vi "Example.vi"() -> ()   [LabVIEW 2019, in "Database_Postgress.lvclass"]
uses:
  Database_Postgress.lvclass
  Query Return.ctl
  Connection Info.ctl
  DatabaseInterface_class/DatabaseInterface.lvclass
panel:
  in  "Query":string="SELECT version();"
  out "Query Return":T1[](array[typedef])
  out "error out":errorcluster
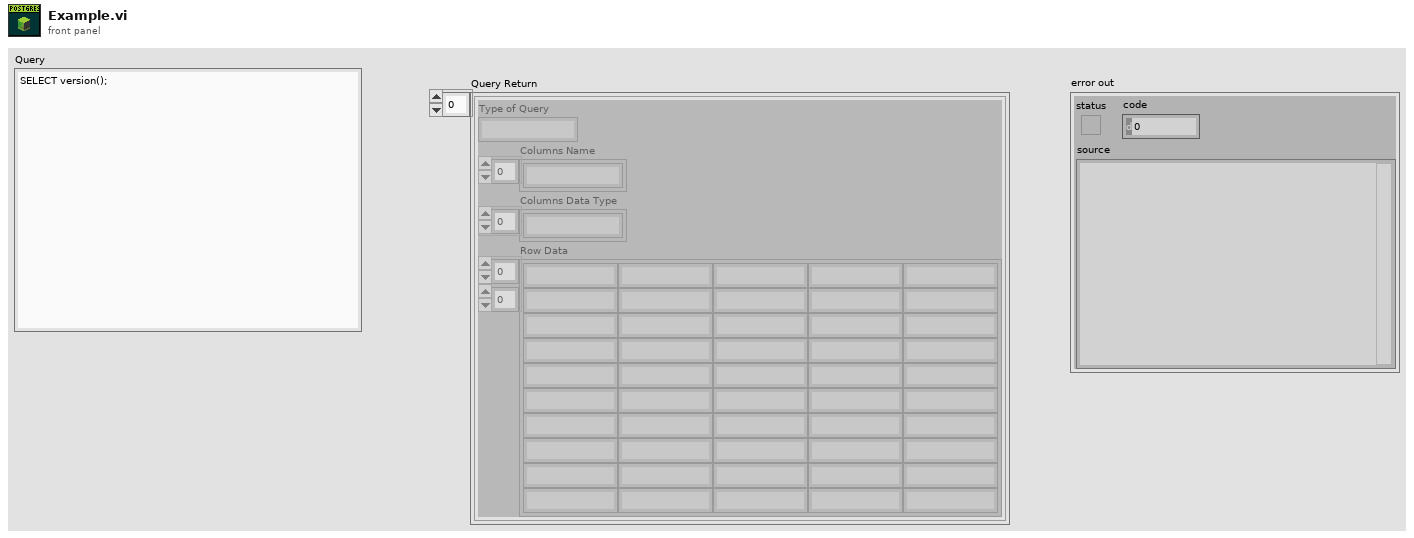
[diagram p1: front panel]
types:
  T1 = typedef "DatabaseInterface.lvclass/Query Return.ctl" = cluster{"Type of Query":string, "Columns Name":string[], "Columns Data Type":string[], "Row Data":string[][]}
  T2 = typedef "DatabaseInterface.lvclass/Connection Info.ctl" = cluster{"IP_Address":string, "Port":u16, "Timeout":i32, "User":string, "Password":string, "Database":string}
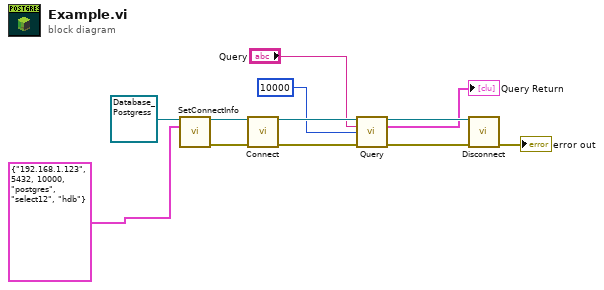
[diagram p0: block diagram]
diagram:
  n1 = call-dynamic "SetConnectInfo.vi"("reference in"=refnum<class "Database_Postgress.lvclass"> refnum, "Connection Info"=T2 {"IP_Address"="192.168.1.123", "Port"=5432, "Timeout"=10000, "User"="postgres", "Password"="select12", "Database"="hdb"}) -> ("reference out"=w12:refnum<class "Database_Postgress.lvclass">, "error out"=w11:errorcluster)  [unwired: 12 in]
  n2 = call-dynamic "Connect.vi"("reference in"=w12, "error in (no error)"=w11) -> ("reference out"=w7:refnum<class "Database_Postgress.lvclass">, "error out"=w8:errorcluster)  [unwired: 12 in]
  n3 = call-dynamic "Query.vi"("reference in"=w7, "Query"="Query", "Timeout"=10000, "error in (no error)"=w8) -> ("reference out"=w5:refnum<class "Database_Postgress.lvclass">, "Query Return"=→"Query Return":T1[], "error out"=w4:errorcluster)  [unwired: 9 in]
  n4 = call-dynamic "Disconnect.vi"("reference in"=w5, "error in (no error)"=w4) -> ("error out"=→"error out":errorcluster)  [unwired: 12 in, 1 out]
